vi "bead_dropper.vi"() -> ()   [LabVIEW 2016]
uses:
  <vilib>/Instr/_visa.llb/VISA Open Access Mode.ctl
panel:
  in  "seconds between steps":u32=5
  out "Last Voltage":dbl=17.5
  in  "stop":bool
  in  "Stop  Frequency (kHz)":dbl=300.0 format="%#.6g"
  in  "Start Frequency (kHz)":dbl=100.0 format="%#.6g"
  in  "Sweep Time (s)":dbl=0.1 format="%#.6g"
  in  "Step size (V)":dbl=0.3
  in  "Start Voltage (V)":dbl=16.0
  in  "Number of steps":i32=30
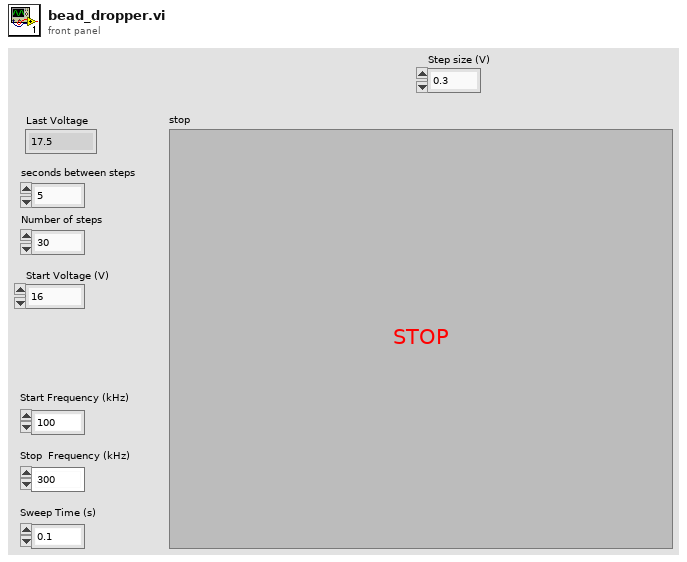
[diagram p1: front panel]
types:
  T1 = typedef "VISA Open Access Mode.ctl" = u32
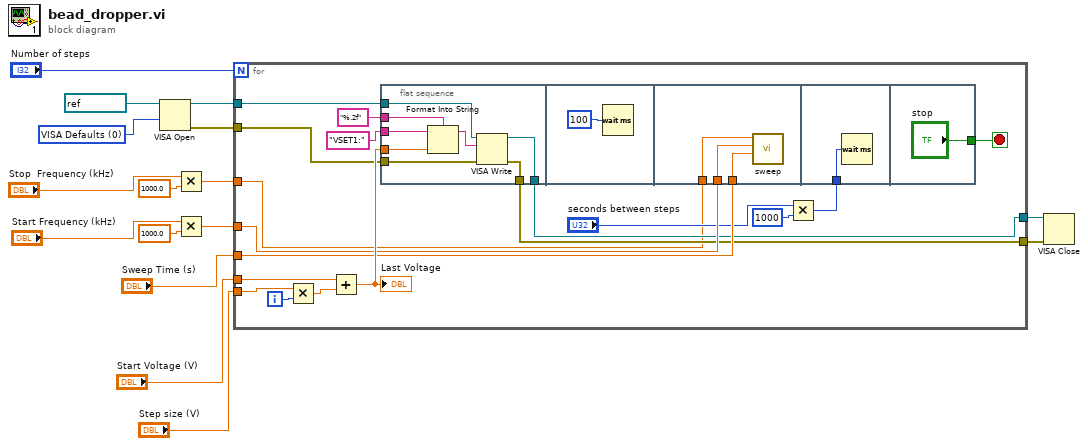
[diagram p0: block diagram]
diagram:
  w15 = T1 0 items=["VISA Defaults"=0, "Exclusive Lock"=1, "Load Configured Settings"=4] ("Access Mode")
  n1 = VISA Open(access mode=w15, VISA resource name=refnum<visa-resource-name> "COM9") -> (VISA resource name=w14:refnum<visa-resource-name>, error out=w12:errorcluster)  [unwired: 3 in]
  n2 = Multiply(x="Stop  Frequency (kHz)", y=1000.0) -> (x*y=w1:dbl)
  n3 = Multiply(x="Start Frequency (kHz)", y=1000.0) -> (x*y=w6:dbl)
  n4 = for {
    N: "Number of steps" -> [_]
    tunnel: "Start Voltage (V)" -> [w34]
    tunnel: "Step size (V)" -> [w33]
    tunnel: w6 -> [w26]
    tunnel: "Sweep Time (s)" -> [w27]
    tunnel: w14 -> [w25]
    tunnel: [w24] -> w13
    tunnel: w12 -> [w23]
    tunnel: [w22] -> w11
    tunnel: w1 -> [w17]
    i -> [w32]
    stop <- w18 stop-if-true
    n5 = Multiply(x=w33, y=w32) -> (x*y=w31:dbl)
    n6 = Add(x=w34, y=w31) -> (x+y=w30:dbl)
    "Last Voltage" <- w30
    n7 = flat-sequence {
      tunnel: w30 -> [w42]
      tunnel: "VSET1:" ("write buffer") -> [w41]
      tunnel: "%.2f" ("format string") -> [w40]
      tunnel: w25 -> [w39]
      tunnel: [w38] -> w24
      tunnel: w23 -> [w37]
      tunnel: [w36] -> w22
      tunnel: w27 -> [w46]
      tunnel: w26 -> [w45]
      tunnel: w17 -> [w44]
      tunnel: w19 -> [w47]
      tunnel: ["stop"] -> w18
      frame #0 {
        n8 = Format Into String(format string=w40, initial string=w41, w42) -> (resulting string=w35:string)  [unwired: 1 in, 1 out]
        n9 = VISA Write(VISA resource name=w39, write buffer=w35, error in (no error)=w37) -> (VISA resource name out=w38:refnum<visa-resource-name>, error out=w36:errorcluster)  [unwired: 1 out]
      }
      frame #1 {
        n10 = Wait (ms)(milliseconds to wait=u32 100) -> ()  [unwired: 1 out]
      }
      frame #2 {
        n11 = call "sweep.vi"("Sweep Time (1.00 s)"=w46, "Start Frequency (100.0 Hz)"=w45, "Stop  Frequency (1000.0 Hz)"=w44) -> ()  [unwired: 9 in]
      }
      frame #3 {
        n12 = Wait (ms)(milliseconds to wait=w47) -> ()  [unwired: 1 out]
      }
      frame #4 {
      }
    }
    n13 = Multiply(x="seconds between steps", y=u32 1000) -> (x*y=w19:u32)
  }
  n14 = VISA Close(VISA resource name=w13, error in (no error)=w11) -> ()  [unwired: 1 out]
